vi "3.1.1-VectorNav.vi"(10 "error in":errorcluster, 11 "FPGA Ref In":T1) -> (1 "Data":dbl[](array[numeric]), 2 "error out":errorcluster, 3 "FPGA VI Reference Out":T1)   [LabVIEW 2010]
uses:
  3.1.1-VectorNav Registers.ctl
  4-High Neurons/4.1-FPGA VI Typedef.ctl
panel:
  in  "Command type":T2(ring)
  out "Register":T3
  out "Header":string
  out "Reading":bool=TRUE
  out "Waiting":bool=TRUE
  out "Writing":bool=TRUE
  out "Reply":string
  in  "Manual command":string="$VNRRG,08*7B"
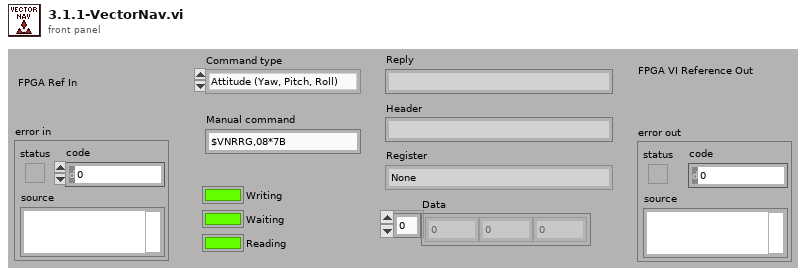
[diagram p1: front panel]
types:
  T1 = typedef "4.1-FPGA VI Typedef.ctl" = refnum<k20>
  T2 = enum16{"Attitude (Yaw, Pitch, Roll)", "Tare", "Manual"}
  T3 = typedef "3.1.1-VectorNav Registers.ctl" = enum16{"None", "Model Number", "Hardware Revision", "Serial Number", "Firmware Version", "Serial Baud Rate", "Async Data Output Type", "Async Data Output Freq", "Attitude (Yaw, Pitch, Roll)", "Attitude (Quaternion)"}
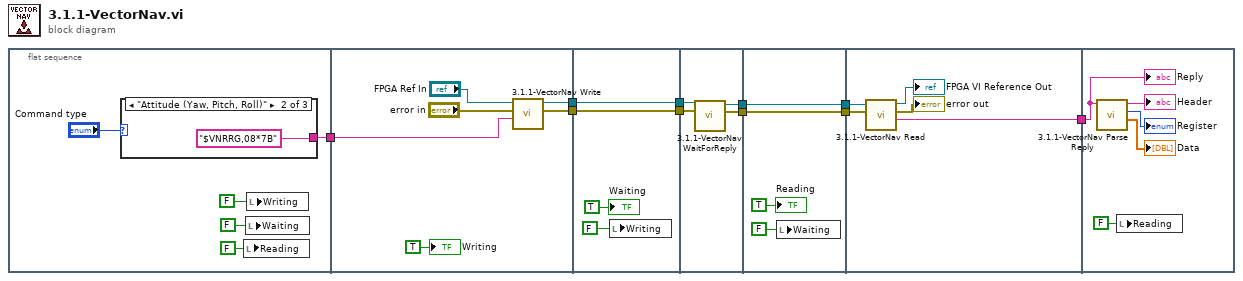
[diagram p0: block diagram]
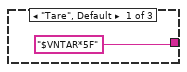
[diagram p2: hidden frame]
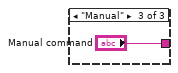
[diagram p3: hidden frame]
diagram:
  n1 = flat-sequence {
    tunnel: [w11] -> w1
    tunnel: [w24] -> w10
    tunnel: [w23] -> w8
    tunnel: w1 -> [w21]
    tunnel: w10 -> [w28]
    tunnel: [w28] -> w9
    tunnel: w8 -> [w27]
    tunnel: [w27] -> w7
    tunnel: w9 -> [w31]
    tunnel: w7 -> [w32]
    tunnel: [w30] -> w6
    tunnel: [w29] -> w4
    tunnel: w6 -> [w36]
    tunnel: [w36] -> w5
    tunnel: w4 -> [w35]
    tunnel: [w35] -> w3
    tunnel: w5 -> [w41]
    tunnel: w3 -> [w40]
    tunnel: [w39] -> w2
    tunnel: w2 -> [w43]
    frame #0 {
      n2 = case shown="\"Attitude (Yaw, Pitch, Roll)\"" "Command type" {
        tunnel: ["$VNTAR*5F" "$VNRRG,08*7B" "Manual command"] -> w11
        frame "Tare", Default {
        }
        frame "Attitude (Yaw, Pitch, Roll)" {
        }
        frame "Manual" {
        }
      }
      n3 = local write "Reading"(FALSE ("Writing")) -> ()
      n4 = local write "Waiting"(FALSE ("Writing")) -> ()
      n5 = local write "Writing"(FALSE ("Writing")) -> ()
    }
    frame #1 {
      n6 = call "3.1.1-VectorNav Write.vi"("Command"=w21, "error in"="error in", "FPGA Ref In"="FPGA Ref In") -> ("error out"=w23:errorcluster, "FPGA VI Reference Out"=w24:T1)  [unwired: 7 in]
      "Writing" <- TRUE
    }
    frame #2 {
      n7 = local write "Writing"(FALSE ("Writing")) -> ()
      "Waiting" <- TRUE
    }
    frame #3 {
      n8 = call "3.1.1-VectorNav WaitForReply.vi"("error in"=w32, "FPGA Ref In"=w31) -> ("error out"=w30:errorcluster, "FPGA VI Reference Out"=w29:T1)  [unwired: 8 in]
    }
    frame #4 {
      n9 = local write "Waiting"(FALSE ("Writing")) -> ()
      "Reading" <- TRUE
    }
    frame #5 {
      n10 = call "3.1.1-VectorNav Read.vi"("error in"=w41, "FPGA Ref In"=w40) -> ("Reply"=w39:string, "error out"=→"error out":errorcluster, "FPGA VI Reference Out"=→"FPGA VI Reference Out":T1)  [unwired: 7 in]
    }
    frame #6 {
      n11 = call "3.1.1-VectorNav Parse Reply.vi"("Input String"=w43) -> ("Data"=→"Data":dbl[], "Register"=→"Register":T3, "Header"=→"Header":string)  [unwired: 8 in]
      n12 = local write "Reading"(FALSE ("Writing")) -> ()
      "Reply" <- w43
    }
  }
